vi "Read IP Filter.vi"(8 "error in (no error)":errorcluster, 11 "L2Enet_RW_CORE in":refnum<class "L2ENET_RW_CORE.lvclass">) -> (0 "error out":errorcluster, 2 "IP Filter":T1[](array[typedef]) {"Protocol" items=["ICMP"=1, "IGMP"=2, "TCP"=6, "UDP"=17]; "Dest IP Address" format="%.0x"; "Source IP Address" format="%.0x"}, 3 "L2Enet_RW_CORE out":refnum<class "L2ENET_RW_CORE.lvclass">)   [LabVIEW 2021, in "L2ENET_RW_CORE.lvclass"]
uses:
  L2ENET_RW_CORE.lvclass
  L2ENET_RW_CORE.lvclass/L2ENET_RW_CORE.ctl
  <vilib>/CIF Foundation/CIF Enet Parse and Build/typedef/L2 & L3/IPV4 Protocol Ring.ctl
  <vilib>/CIF Foundation/CIF Enet Parse and Build/Ethernet_Parse_Build_CIF.lvlib
  <vilib>/CIF Foundation/CIF Enet Parse and Build/typedef/L2 & L3/IPV4 Filter.ctl
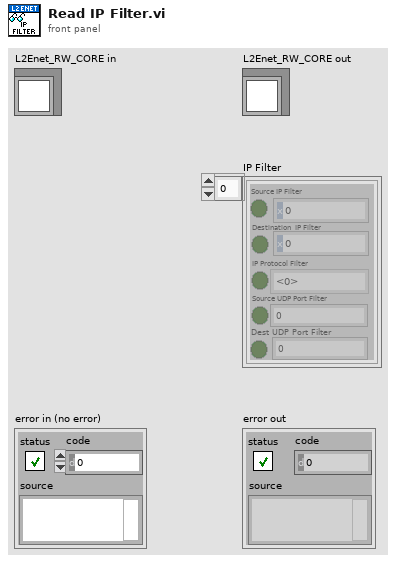
[diagram p1: front panel]
types:
  T1 = typedef "Ethernet_Parse_Build_CIF.lvlib/IPV4 Filter.ctl" = cluster{"Source IP Filter":bool, "Source IP Address":u32, "Destination  IP Filter":bool, "Dest IP Address":u32, "IP Protocol Filter":bool, "Protocol":T2, "Source UDP Port Filter":bool, "UDP Source Port":u16, "Dest UDP Port Filter ":bool, "UDP Dest Port":u16}
  T2 = typedef "Ethernet_Parse_Build_CIF.lvlib/IPV4 Protocol Ring.ctl" = u8
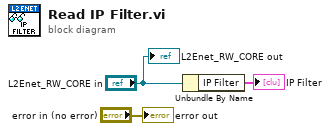
[diagram p0: block diagram]
diagram:
  n1 = Unbundle By Name("L2Enet_RW_CORE in") -> ("IP Filter"=→"IP Filter":T1[])
  "error out" <- "error in (no error)"
  "L2Enet_RW_CORE out" <- "L2Enet_RW_CORE in"
